vi "Create REST Client (plugin).vi"(4 "Default Headers ([JSON])":cluster{"header":string, "value":string}[](array[cluster])=[{"header"="Content-Type", "value"="application/json"}], 5 "http-client (default)":refnum<class "http-client.lvclass">, 6 "Verify Server(true)":bool=TRUE, 7 "Cookie File":path, 8 "error in (no error)":errorcluster, 9 "Authentication":cluster{"Username":string, "Password":string}, 10 "Escape URLs (true)":bool=TRUE, 11 "Base URL":string) -> (0 "error out":errorcluster, 3 "REST Client out":refnum<class "REST Client.lvclass">)   [LabVIEW 2020, in "REST Client.lvlib" / "REST Client.lvclass"]
doc: "The VI provides multiple arguments for defining how to create the JKI REST Client instance.\n\n<b>Base URL</b> specifies the base URL to be used for the HTTP requests.\n\n<b>Escape URLs</b> when true instruct the REST Client to escape all URLs before executing the requests. If you have already escaped the URLs, set this to false.\n\n<b>Authentication</b> allows setting the username and password for services that use HTTP authentication.\n\n<b>Verify Server</b> when true instructs the REST Client to validate the certificate of the server when HTTPS protocol is being used.\n\n<b>Default Headers</b> specifies an array of headers to be used with every requests. Defaults to application/json content type.\n\n<b>Cookie File</b> specifies a file path to be used for cookies."
uses:
  REST Client.lvclass
  REST Client.lvclass/REST Client.ctl
  http-client/http-client.lvclass
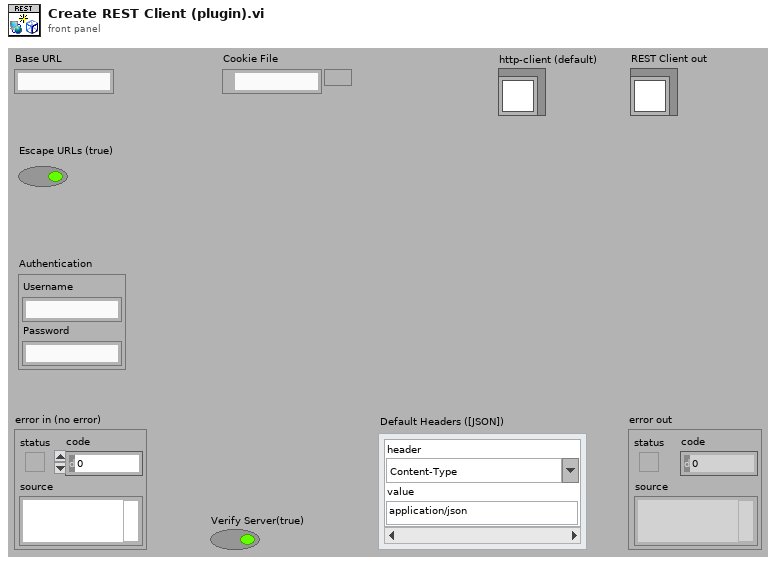
[diagram p1: front panel]
types:
  T1 = cluster{"http-client out":refnum<class "http-client.lvclass">, "Default Headers ([JSON])":cluster{"header":string, "value":string}[]}
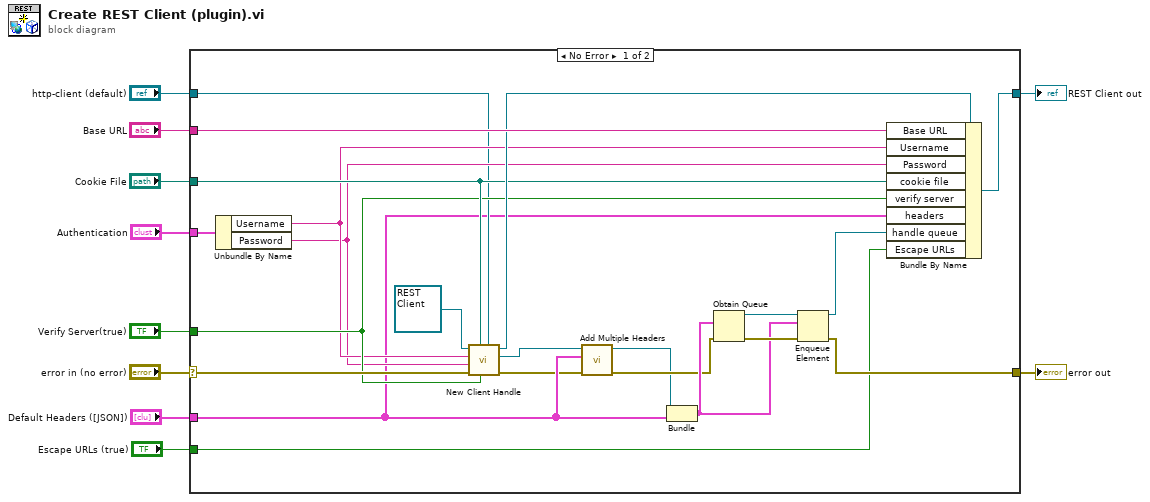
[diagram p0: block diagram]
diagram:
  n1 = case shown="No Error" "error in (no error)" {
    selector: "error in (no error)" -> [w30 w33]
    tunnel: [w24 w33] -> w9
    tunnel: [w32 _] -> w7
    tunnel: "http-client (default)" -> [w17 _]
    tunnel: "Cookie File" -> [w28 _]
    tunnel: "Verify Server(true)" -> [w27 _]
    tunnel: "Default Headers ([JSON])" -> [w14 _]
    tunnel: "Authentication" -> [w20 _]
    tunnel: "Base URL" -> [w31 _]
    tunnel: "Escape URLs (true)" -> [w21 _]
    frame No Error {
      n2 = Unbundle By Name(w20) -> ("Username"=w19:string, "Password"=w18:string)
      n3 = call "New Client Handle.vi"("http-client (default)"=w17, "verify server(true)"=w27, "cookie file"=w28, "error in (no error)"=w30, "password"=w18, "username"=w19, "REST Client in"=refnum<class "REST Client.lvclass"> refnum) -> ("error out"=w13:errorcluster, "http-client"=w15:refnum<class "http-client.lvclass">, "REST Client out"=w29:refnum<class "REST Client.lvclass">)  [unwired: 2 in]
      n4 = call "Add Multiple Headers.vi"("error in"=w13, "headers"=w14, "http-client in"=w15) -> ("error out"=w12:errorcluster, "http-client out"=w11:refnum<class "http-client.lvclass">)  [unwired: 7 in]
      n5 = Bundle("http-client out"=w11, "Default Headers ([JSON])"=w14) -> (w23:T1)  [unwired: 1 in]
      n6 = Obtain Queue(element data type=w23, error in (no error)=w12) -> (queue out=w26:refnum<queue>, error out=w25:errorcluster)  [unwired: 3 in, 1 out]
      n7 = Enqueue Element(queue=w26, element=w23, error in (no error)=w25) -> (queue out=w22:refnum<queue>, error out=w24:errorcluster)  [unwired: 1 in, 1 out]
      n8 = Bundle By Name(cluster=w29, "Base URL"=w31, "Username"=w19, "Password"=w18, "cookie file"=w28, "verify server"=w27, "headers"=w14, "handle queue"=w22, "Escape URLs"=w21) -> (w32:refnum<class "REST Client.lvclass">)
    }
    frame Error {
    }
  }
  "error out" <- w9
  "REST Client out" <- w7
